vi "ZCAN_ResetCAN.vi"(8 "error in (no error)":errorcluster caption="错误输入（无错误）", 10 "can_handle":u32) -> (0 "error out":errorcluster caption="错误输出", 2 "reset_success?":bool)   [LabVIEW 2021, in "zlgcan.lvlib"]
doc: "该函数用于复位CAN通道，释放通道句柄。\n\n可通过ZCAN_StartCAN重新获取通道句柄。"
uses:
  zlgcan.lvlib
  <userlib>/zlg/zlgcan_wrap.dll
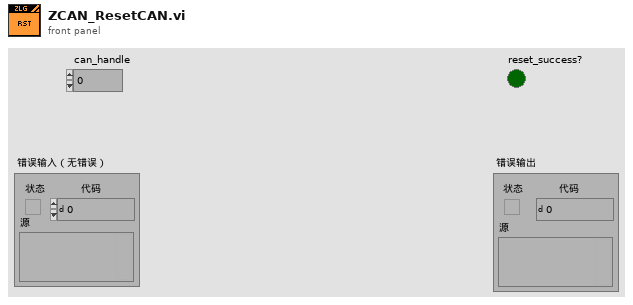
[diagram p1: front panel]
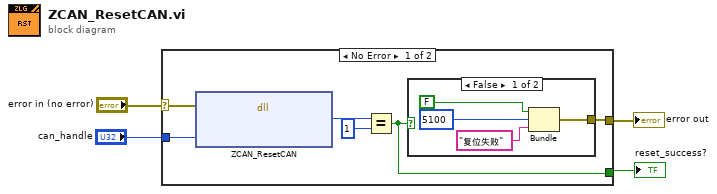
[diagram p0: block diagram]
diagram:
  n1 = case shown="No Error" "error in (no error)" {
    selector: "error in (no error)" -> [w10 w15]
    tunnel: [w7 w15] -> w3
    tunnel: "can_handle" -> [w9 _]
    tunnel: [w5 _] -> w1
    frame No Error {
      n2 = dll-call lib="C:/Program Files (x86)/National Instruments/LabVIEW 2021/user.lib/zlg/zlgcan_wrap.dll" fn="ZCAN_ResetCAN"(error in=w10, "can_handle"=w9) -> ("return"=w6:u32)  [unwired: 3 in, 2 out]
      n3 = Equal?(x=w6, y=u32 1) -> (x = y?=w5:bool)
      n4 = case shown="False" w5 {
        tunnel: [w11 _] -> w7
        frame False {
          n5 = Bundle("status"=FALSE, "code"=5100, "消息"="复位失败") -> (w11:cluster{"status":bool, "code":i32, "消息":string})  [unwired: 1 in]
        }
        frame True {
        }
      }
    }
    frame Error {
    }
  }
  "error out" <- w3
  "reset_success?" <- w1
